vi "Read Waveforms (Multiple).vi"(8 "error in (no error)":errorcluster, 9 "Timeout (10000 ms)":u32=10000, 10 "Channels":i32[](array[ring]) items=["Channel 1"=0, "Channel 2"=1, "Channel 3"=2, "Channel 4"=3, "Waveform Memory 1"=5, "Waveform Memory 2"=6, "Serial Bus 1"=7, "Serial Bus 2"=8, "Digital Bus Low"=9, "Digital Bus High "=10, "Digital Bus 1"=11, "Digital Bus 2"=12, "External"=29, "Function 1"=32, "Function 2"=33, "Function 3"=34, "Function 4"=35, "Math 1"=36, "Math 2"=37, "Math 3"=38, "Math 4"=39, "FFT"=40, "Analog Bus"=41], 11 "VISA resource name":refnum<visa-resource-name>) -> (0 "error out":errorcluster, 2 "Waveform Data":waveform(dbl)[](graph), 3 "VISA resource name out":refnum<visa-resource-name>)   [LabVIEW 2015, in "Agilent 2000 3000 X-Series.lvlib"]
doc: "Initiates an acquisition on all channels that you enabled with the Configure Channel VI. The VI waits for the acquisition to complete and returns the waveform for the <B>Source Channel</B> you specified. If the oscilloscope did not complete the acquisition within the time period you specify with the <B>Timeout</B> control, the VI returns a timeout error. A common cause for a timeout error is the acquisition was not triggered. For example, the trigger level is out of range of the waveform. \n\n<B>Note(s):</B> \nIf your instrument does not support auto compensation for probe attenuation, you may need to adjust the scaling of the waveform data accordingly. This is handled automatically in the Configure Channel VI or can be done manually by multiplying the waveform data by the probe attenuation."
uses:
  Agilent 2000 3000 X-Series.lvlib
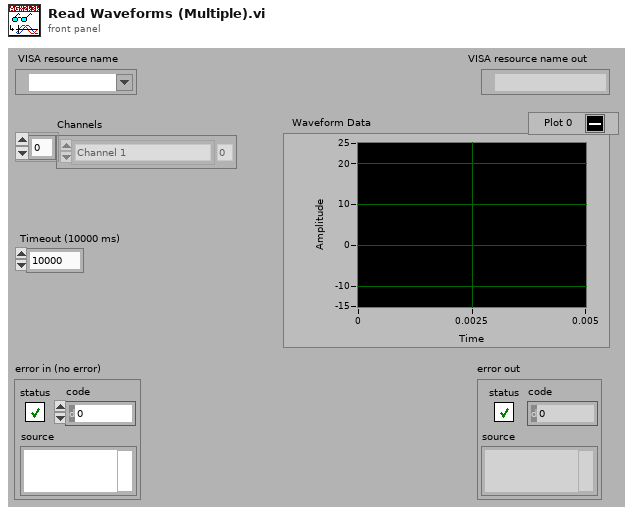
[diagram p1: front panel]
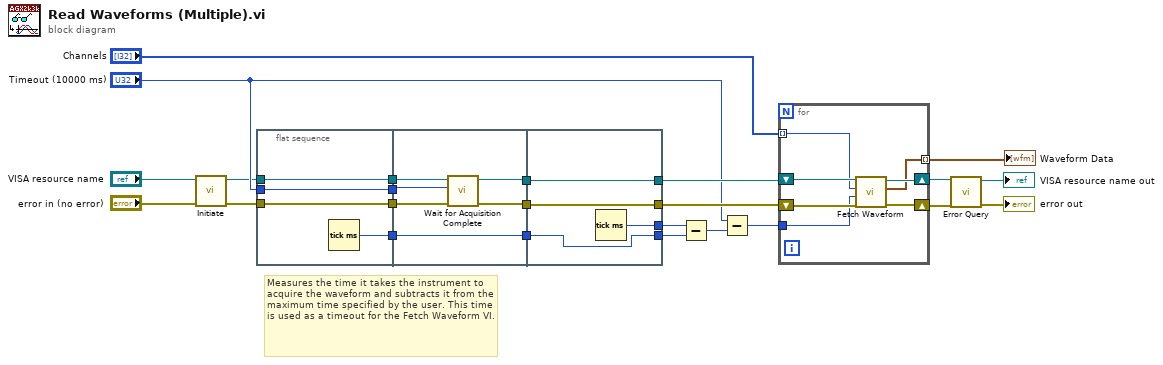
[diagram p0: block diagram]
diagram:
  # "Measures the time it takes the instrument to acquire the waveform and subtracts it from the maximum time specified by the user. This time is used as a timeout for the Fetch Waveform VI."
  n1 = call "Initiate.vi"("error in (no error)"="error in (no error)", "VISA resource name"="VISA resource name") -> ("error out"=w12:errorcluster, "VISA resource name out"=w11:refnum<visa-resource-name>)  [unwired: 8 out]
  n2 = flat-sequence {
    tunnel: w11 -> [w27]
    tunnel: [w27] -> w7
    tunnel: w12 -> [w26]
    tunnel: [w26] -> w6
    tunnel: "Timeout (10000 ms)" -> [w25]
    tunnel: [w25] -> w5
    tunnel: [w28] -> w4
    tunnel: w7 -> [w34]
    tunnel: [w31] -> w3
    tunnel: w6 -> [w33]
    tunnel: [w30] -> w2
    tunnel: w5 -> [w32]
    tunnel: w4 -> [w29]
    tunnel: [w29] -> w1
    tunnel: [w37] -> w19
    tunnel: w3 -> [w37]
    tunnel: [w36] -> w18
    tunnel: w2 -> [w36]
    tunnel: [w35] -> w21
    tunnel: w1 -> [w35]
    tunnel: [w38] -> w20
    frame #0 {
      n3 = Tick Count (ms)() -> (millisecond timer value=w28:u32)
    }
    frame #1 {
      n4 = call "Wait for Acquisition Complete.vi"("error in (no error)"=w33, "Maximum Time (10000)"=w32, "VISA resource name"=w34) -> ("error out"=w30:errorcluster, "VISA resource name out"=w31:refnum<visa-resource-name>)  [unwired: 7 out]
    }
    frame #2 {
      n5 = Tick Count (ms)() -> (millisecond timer value=w38:u32)
    }
  }
  n6 = Subtract(x=w20, y=w21) -> (x-y=w22:u32)
  n7 = Subtract(x="Timeout (10000 ms)", y=w22) -> (x-y=w17:u32)
  n8 = for {
    shift-right: [w42] -> w8
    shift-left: w18 -> [w41]
    tunnel: "Channels" -> [w39] mode=indexing
    tunnel: [w43] -> w10 mode=indexing
    shift-right: [w44] -> w9
    shift-left: w19 -> [w45]
    tunnel: w17 -> [w40]
    n9 = call "Fetch Waveform.vi"("error in (no error)"=w41, "Timeout (10000)"=w40, "Source Channel (0: Channel 1)"=w39, "VISA resource name"=w45) -> ("error out"=w42:errorcluster, "Waveform Data"=w43:waveform(dbl), "VISA resource name out"=w44:refnum<visa-resource-name>)  [unwired: 1 in, 4 out]
  }
  "Waveform Data" <- w10
  n10 = call "Error Query.vi"("error in (no error)"=w8, "VISA resource name"=w9) -> ("error out"=→"error out":errorcluster, "VISA resource name out"=→"VISA resource name out":refnum<visa-resource-name>)  [unwired: 8 out]
